vi "second_gate_controller.vi"(10 "Numerical Argument":dbl, 11 "Command":T1(ring)=enum."Read Voltage") -> (3 "Response":string)   [LabVIEW 2021]
panel:
  # "SECOND GATE CONTROLLER"
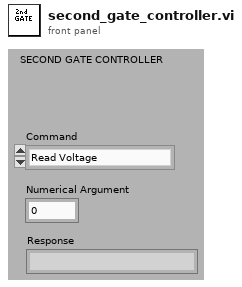
[diagram p1: front panel]
types:
  T1 = enum16{"Set Voltage", "Read Voltage", "Read Current", "Output On", "Output Off", "Set Increment", "Set Increment Time", "Stop Voltage Set"}
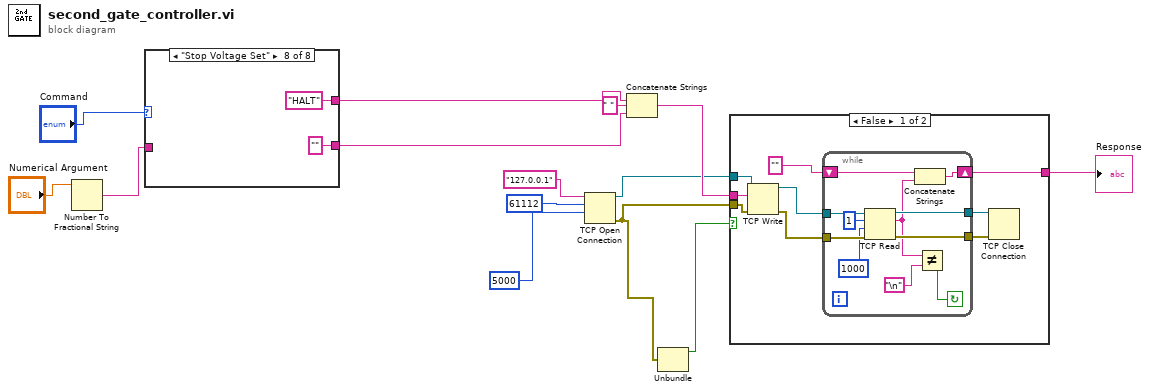
[diagram p0: block diagram]
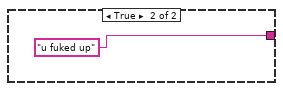
[diagram p2: hidden frame]
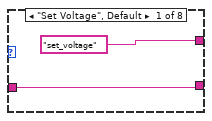
[diagram p3: hidden frame]
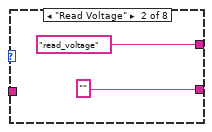
[diagram p4: hidden frame]
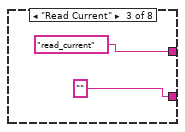
[diagram p5: hidden frame]
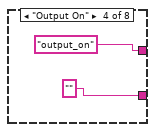
[diagram p6: hidden frame]
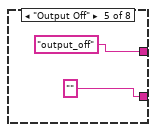
[diagram p7: hidden frame]
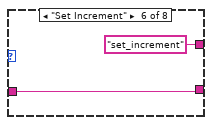
[diagram p8: hidden frame]
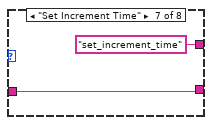
[diagram p9: hidden frame]
diagram:
  n1 = Number To Fractional String(number="Numerical Argument") -> (F-format string=w8:string)  [unwired: 3 in]
  n2 = case shown="\"Stop Voltage Set\"" "Command" {
    tunnel: ["set_voltage" ("data in") "read_voltage" ("data in") "read_current" ("data in") "output_on" ("data in") "output_off" ("data in") "set_increment" ("data in") "set_increment_time" ("data in") "HALT" ("data in")] -> w12
    tunnel: [w15 "" ("string") "" ("string") "" ("string") "" ("string") w26 w28 "" ("string")] -> w9
    tunnel: w8 -> [w15 _ _ _ _ w26 w28 _]
    frame "Set Voltage", Default {
    }
    frame "Read Voltage" {
    }
    frame "Read Current" {
    }
    frame "Output On" {
    }
    frame "Output Off" {
    }
    frame "Set Increment" {
    }
    frame "Set Increment Time" {
    }
    frame "Stop Voltage Set" {
    }
  }
  n3 = TCP Open Connection(address="127.0.0.1", remote port or service name=u16 61112, timeout ms (60000)=5000) -> (connection ID=w1:refnum<k5>, error out=w3:errorcluster)  [unwired: 2 in]
  n4 = Concatenate Strings(w12, " " ("string"), w9) -> (w2:string)
  n5 = Unbundle(w3) -> ("status"=w4:bool)  [unwired: 2 out]
  n6 = case shown="False" w4 {
    tunnel: [w36 "u fuked up"] -> w5
    tunnel: w3 -> [w35 _]
    tunnel: w2 -> [w34 _]
    tunnel: w1 -> [w33 _]
    frame False {
      n7 = TCP Write(connection ID=w33, data in=w34, error in (no error)=w35) -> (connection ID out=w31:refnum<k5>, error out=w32:errorcluster)  [unwired: 1 in, 1 out]
      n8 = while {
        tunnel: w32 -> [w50]
        tunnel: w31 -> [w49]
        tunnel: [w48] -> w39
        tunnel: [w47] -> w38
        shift-right: [w43] -> w36
        shift-left: "" ("string") -> [w44]
        stop <- w42 continue-if-true
        n9 = TCP Read(connection ID=w49, bytes to read=1, error in (no error)=w50, 9:1000 ("timeout ms (25000)")) -> (connection ID out=w47:refnum<k5>, data out=w41:string, error out=w48:errorcluster)  [unwired: 1 in]
        n10 = Concatenate Strings(w44, w41) -> (w43:string)
        n11 = Not Equal?(x=w41, y="\n") -> (x != y?=w42:bool)
      }
      n12 = TCP Close Connection(connection ID=w38, error in (no error)=w39) -> ()  [unwired: 1 in, 2 out]
    }
    frame True {
    }
  }
  "Response" <- w5
